vi "Queue Comms Enqueue.vi"(8 "error in (no error)":errorcluster, 11 "element":T1) -> (0 "error out":errorcluster)   [LabVIEW 2018, in "PC UDP Writer.lvlib"]
doc: "This subVI enqueues an element in to the communications queue to be handled"
uses:
  PC UDP Writer.lvlib
  Private Controls/Module Data.ctl
  Private Controls/Module Action.ctl
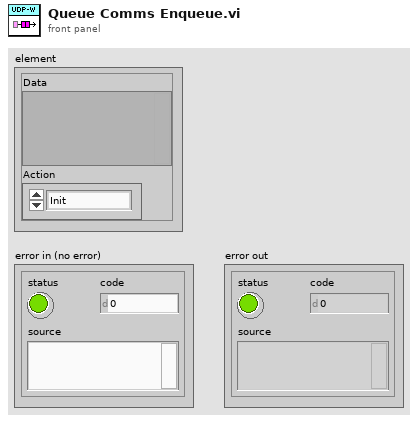
[diagram p1: front panel]
types:
  T1 = typedef "PC UDP Writer.lvlib/Module Data.ctl" = cluster{"Data":variant, "Action":T2}
  T2 = typedef "PC UDP Writer.lvlib/Module Action.ctl" = enum8{"Init", "Waterfall Select", "Bleed Fuel", "Fuel Pressure Reg", "ECS Demand", "Accel Sensitivities", "Accel Filters", "Shunt Relay", "APU Setup", "APU and ECU Control", "APU Start", "Write", "Error", "Exit"}
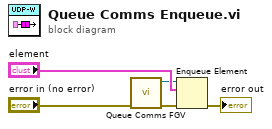
[diagram p0: block diagram]
diagram:
  n1 = call "Queue Comms FGV.vi"("error in (no error)"="error in (no error)") -> ("error out"=w4:errorcluster, "Queue out"=w2:refnum<queue>)  [unwired: 9 in]
  n2 = Enqueue Element(queue=w2, element="element", error in (no error)=w4) -> (error out=→"error out":errorcluster)  [unwired: 1 in, 2 out]
